vi "osciloscope-2-chan.vi"() -> ()   [LabVIEW 2023]
uses:
  <vilib>/Analysis/2dsp.llb/Decimate (single shot, DBL).vi
  <vilib>/express/express analysis/Spectral/Block/exnSpectralBlock spectral measurements peak poly.vi
  <vilib>/express/express analysis/Spectral/Block/exnSpectralBlock spectral measurements peak WFM.vi
  <vilib>/express/express analysis/Spectral/XNode/ExpressSpectralMeasurementsBlockNode.xnode
  <vilib>/Instr/_visa.llb/VISA Configure Serial Port (Instr).vi
  <vilib>/Analysis/NI_AALPro.lvlib
panel:
  in  "Decimation Factor":u8=1 min=1 max=100
  out "Time Domain Indicator":u32
  out "Frerquency Domain Indicator":u32
  in  "Refresh Button":bool
  in  "Frequency Domain (Block Size)":u16(knob) scale=4.0..10.0
  in  "Time Domain (Block Size)":u16(knob) scale=4.0..10.0
  in  "Sampling Frequency (Hz)":sgl
  in  "Stop Button":bool
  in  "COM Port":refnum<visa-resource-name>
  in  "Baud Rate (BPS)":u32=9600
  out "Frequency Domain":cluster{"f0":dbl, "df":dbl, "magnitude":dbl[]}[](graph)
  out "Time Domain":waveform(dbl)[](graph)
  # "2-CHANNEL OSCILOSCOPE"
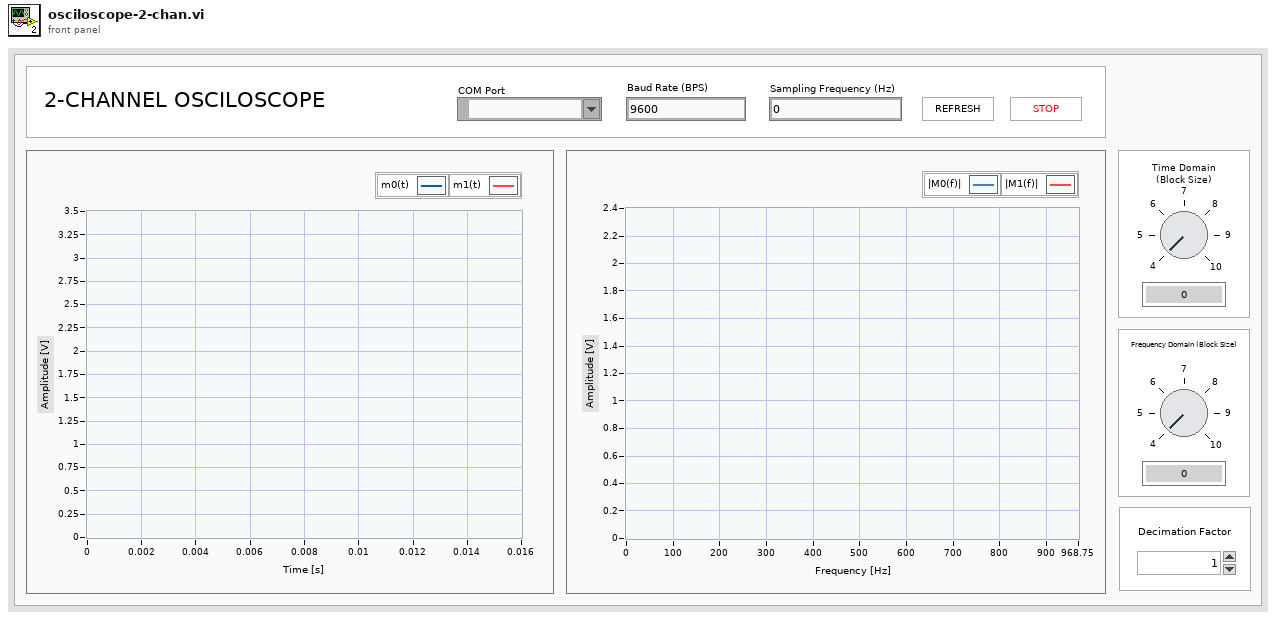
[diagram p1: front panel]
types:
  T1 = cluster{"averaging mode":u16, "weighting mode":u16, "number of averages":u32}
  T2 = cluster{"dB On (F)":bool, "unwrap phase (F)":bool, "convert to degree (F)":bool}
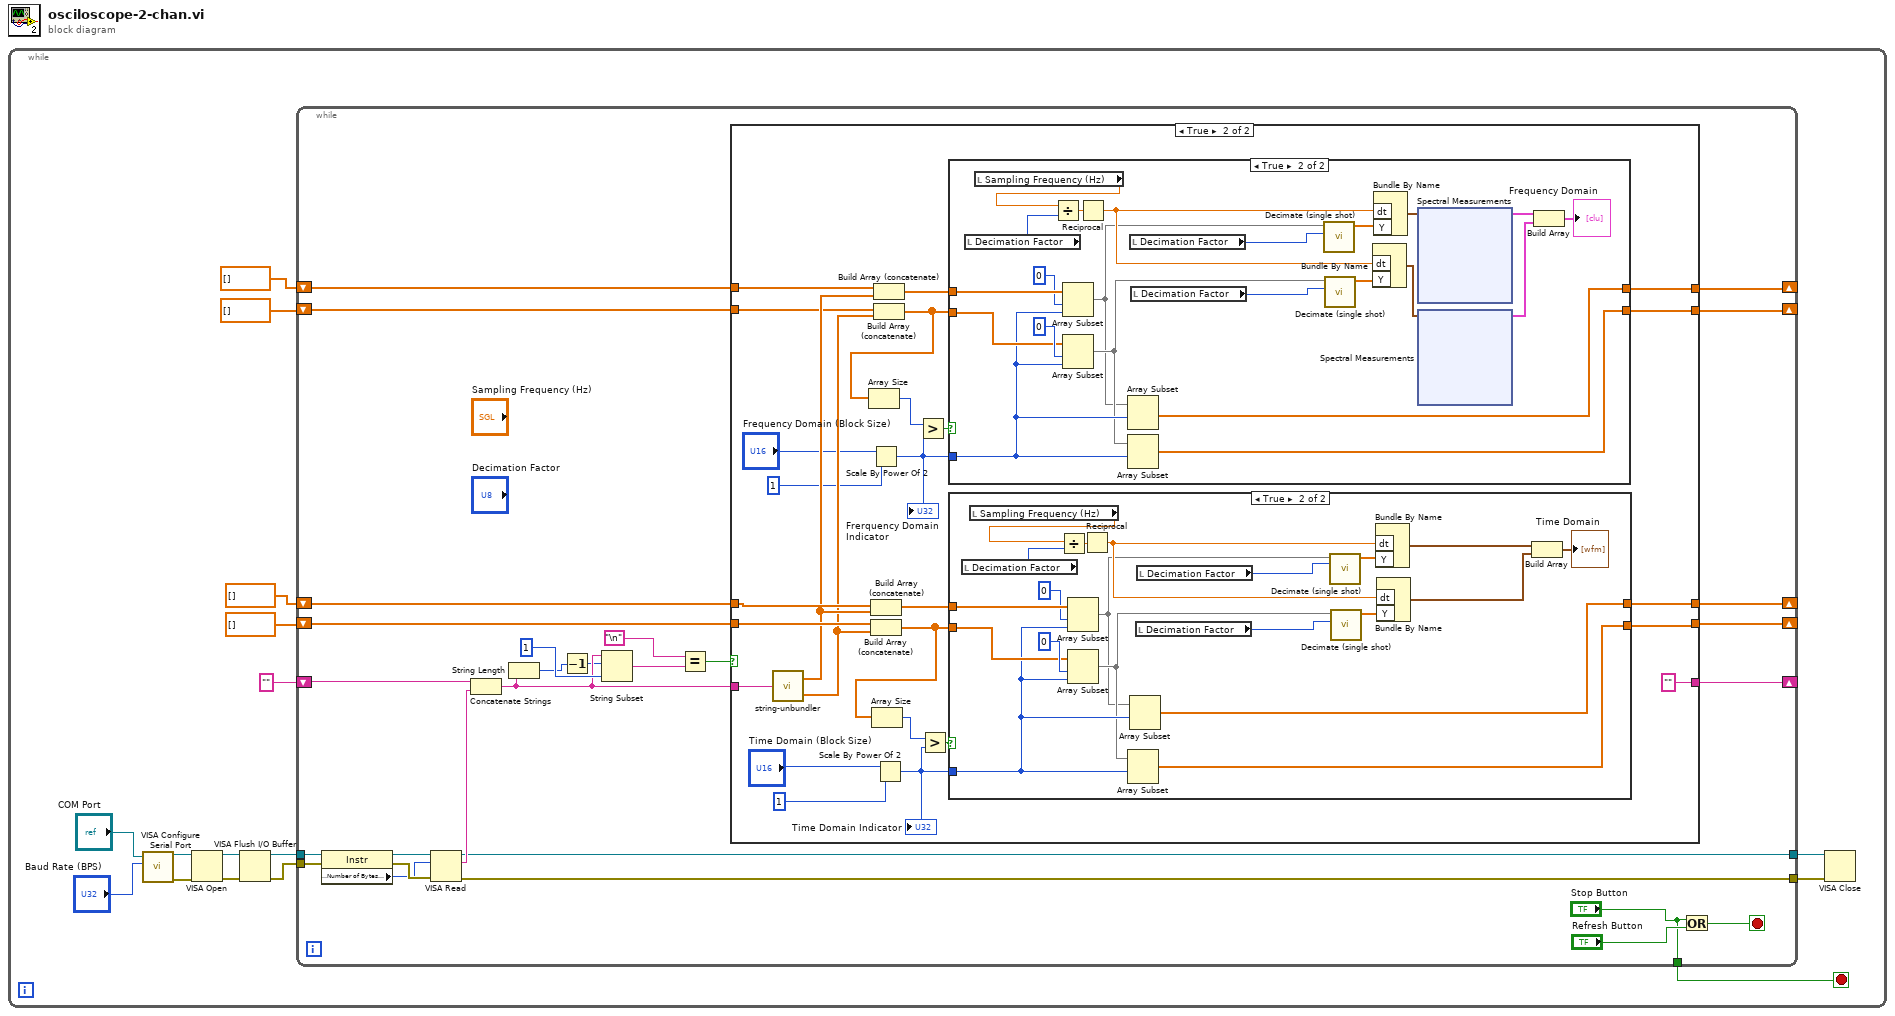
[diagram p0: block diagram]
diagram:
  n1 = while {
    stop <- w1 stop-if-true
    n2 = call-poly "VISA Configure Serial Port"("VISA resource name"="COM Port", "baud rate (9600)"="Baud Rate (BPS)") -> ("VISA resource name out"=w14:refnum<visa-resource-name>, "error out"=w15:errorcluster)  [unwired: 12 in]
    n3 = VISA Open(error in (no error)=w15, VISA resource name=w14) -> (VISA resource name=w13:refnum<visa-resource-name>, error out=w12:errorcluster)  [unwired: 3 in]
    n4 = VISA Flush I/O Buffer(VISA resource name=w13, error in (no error)=w12) -> (VISA resource name out=w16:refnum<visa-resource-name>, error out=w9:errorcluster)  [unwired: 1 in]
    n5 = while {
      tunnel: w16 -> [w44]
      tunnel: w9 -> [w43]
      tunnel: [w24] -> w8
      tunnel: [w25] -> w7
      shift-right: [w37] -> _
      shift-left: "" -> [w38]
      shift-right: [w27] -> _
      shift-left: dbl[] [] -> [w28]
      shift-right: [w26] -> _
      shift-left: dbl[] [] -> [w29]
      shift-right: [w21] -> _
      shift-left: dbl[] [] -> [w23]
      shift-right: [w20] -> _
      shift-left: dbl[] [] -> [w22]
      tunnel: ["Stop Button"] -> w1
      stop <- w19 stop-if-true
      n6 = property class="Instr"(reference=w44, error in=w43) -> (reference out=w42:refnum<visa-resource-name>, error out=w41:errorcluster, "Serial Settings:Number of Bytes at Serial Port"=w40:u32)
      n7 = VISA Read(VISA resource name=w42, byte count=w40, error in (no error)=w41) -> (VISA resource name out=w25:refnum<visa-resource-name>, read buffer=w39:string, error out=w24:errorcluster)  [unwired: 1 out]
      n8 = Concatenate Strings(w38, w39) -> (w35:string)
      n9 = String Length(string=w35) -> (length=w33:i32)
      n10 = Decrement(x=w33) -> (x-1=w34:i32)
      n11 = String Subset(string=w35, offset (0)=w34, length (rest)=1 ("length (rest)")) -> (substring=w31:string)
      n12 = Equal?(x="\n", y=w31) -> (x = y?=w30:bool)
      n13 = case shown="True" w30 {
        tunnel: w29 -> [w48 w74]
        tunnel: w35 -> [w49 w73]
        tunnel: [w49 ""] -> w37
        tunnel: w28 -> [w47 w71]
        tunnel: [w47 w68] -> w27
        tunnel: [w48 w69] -> w26
        tunnel: w23 -> [w46 w63]
        tunnel: w22 -> [w45 w62]
        tunnel: [w46 w61] -> w21
        tunnel: [w45 w60] -> w20
        frame False {
        }
        frame True {
          n14 = call "string-unbundler.vi"("String"=w73) -> ("Array 1"=w65:dbl[], "Array 2"=w64:dbl[])
          n15 = Scale By Power Of 2(n="Frequency Domain (Block Size)", x=u32 1) -> (x*2^n=w54:u32)
          "Frerquency Domain Indicator" <- w54
          n16 = Build Array (concatenate)(w74, w65) -> (w59:dbl[])
          n17 = Build Array (concatenate)(w71, w64) -> (w67:dbl[])
          n18 = Array Size(array=w67) -> (size(s)=w75:i32)
          n19 = Build Array (concatenate)(w63, w65) -> (w66:dbl[])
          n20 = Build Array (concatenate)(w62, w64) -> (w57:dbl[])
          n21 = Array Size(array=w57) -> (size(s)=w56:i32)
          n22 = Scale By Power Of 2(n="Time Domain (Block Size)", x=u32 1) -> (x*2^n=w51:u32)
          "Time Domain Indicator" <- w51
          n23 = Greater?(x=w56, y=w54) -> (0:w58:bool)
          n24 = Greater?(x=w75, y=w51) -> (0:w70:bool)
          n25 = case shown="True" w58 {
            tunnel: w66 -> [w77 w99]
            tunnel: w57 -> [w76 w96]
            tunnel: w54 -> [_ w94]
            tunnel: [w77 w93] -> w61
            tunnel: [w76 w92] -> w60
            frame False {
            }
            frame True {
              n26 = local read "Decimation Factor"() -> (w81:u8)
              n27 = local read "Sampling Frequency (Hz)"() -> (w80:sgl)
              n28 = Divide(x=w80, y=w81) -> (x/y=w82:sgl)
              n29 = Array Subset(array=w99, index=0, length=w94) -> (w83:dbl[])
              n30 = Array Subset(array=w96, index=0, length=w94) -> (w86:dbl[])
              n31 = Reciprocal(x=w82) -> (1/x=w95:sgl)
              n32 = Array Subset(array=w83, index=w94) -> (w93:dbl[])  [unwired: 1 in]
              n33 = Array Subset(array=w86, index=w94) -> (w92:dbl[])  [unwired: 1 in]
              n34 = local read "Decimation Factor"() -> (w79:u8)
              n35 = local read "Decimation Factor"() -> (w78:u8)
              n36 = call-poly <vilib>:"Decimate (single shot).vi"("decimating factor"=w79, "X"=w83) -> ("Decimated Array"=w84:dbl[])  [unwired: 8 in, 1 out]
              n37 = call-poly <vilib>:"Decimate (single shot).vi"("decimating factor"=w78, "X"=w86) -> ("Decimated Array"=w85:dbl[])  [unwired: 8 in, 1 out]
              n38 = Bundle By Name("dt"=w95, "Y"=w85) -> (w88:waveform(dbl))  [unwired: 1 in]
              n39 = Bundle By Name("dt"=w95, "Y"=w84) -> (w87:waveform(dbl))  [unwired: 1 in]
              n40 = xnode "Spectral Measurements"("Signals"=w87) -> ("FFT - (Peak)"=w89:cluster{"f0":dbl, "df":dbl, "magnitude":dbl[]})  [unwired: 1 in, 2 out]
              n41 = xnode "Spectral Measurements"("Signals"=w88) -> ("FFT - (Peak)"=w90:cluster{"f0":dbl, "df":dbl, "magnitude":dbl[]})  [unwired: 1 in, 2 out]
              n42 = Build Array(w89, w90) -> (→"Frequency Domain":cluster{"f0":dbl, "df":dbl, "magnitude":dbl[]}[])
            }
          }
          n43 = case shown="True" w70 {
            tunnel: w59 -> [w121 w141]
            tunnel: w67 -> [w120 w139]
            tunnel: w51 -> [_ w134]
            tunnel: [w121 w133] -> w69
            tunnel: [w120 w132] -> w68
            frame False {
            }
            frame True {
              n44 = local read "Decimation Factor"() -> (w126:u8)
              n45 = local read "Sampling Frequency (Hz)"() -> (w125:sgl)
              n46 = Divide(x=w125, y=w126) -> (x/y=w124:sgl)
              n47 = Array Subset(array=w141, index=0, length=w134) -> (w129:dbl[])
              n48 = Array Subset(array=w139, index=0, length=w134) -> (w131:dbl[])
              n49 = Reciprocal(x=w124) -> (1/x=w135:sgl)
              n50 = Array Subset(array=w131, index=w134) -> (w132:dbl[])  [unwired: 1 in]
              n51 = Array Subset(array=w129, index=w134) -> (w133:dbl[])  [unwired: 1 in]
              n52 = local read "Decimation Factor"() -> (w122:u8)
              n53 = local read "Decimation Factor"() -> (w123:u8)
              n54 = call-poly <vilib>:"Decimate (single shot).vi"("decimating factor"=w123, "X"=w129) -> ("Decimated Array"=w128:dbl[])  [unwired: 8 in, 1 out]
              n55 = call-poly <vilib>:"Decimate (single shot).vi"("decimating factor"=w122, "X"=w131) -> ("Decimated Array"=w130:dbl[])  [unwired: 8 in, 1 out]
              n56 = Bundle By Name("dt"=w135, "Y"=w128) -> (w136:waveform(dbl))  [unwired: 1 in]
              n57 = Bundle By Name("dt"=w135, "Y"=w130) -> (w137:waveform(dbl))  [unwired: 1 in]
              n58 = Build Array(w136, w137) -> (→"Time Domain":waveform(dbl)[])
            }
          }
        }
      }
      n59 = Or(x="Stop Button", y="Refresh Button") -> (x .or. y?=w19:bool)
    }
    n60 = VISA Close(VISA resource name=w7, error in (no error)=w8) -> ()  [unwired: 1 out]
  }
